vi "NMEA serial.vi"() -> ()   [LabVIEW 2016, in "AIRMAR WeatherCaster.lvlib"]
uses:
  AIRMAR WeatherCaster.lvlib
  NMEA_WIMDA-data.ctl
  NMEA_GPRMC-data.ctl
  NMEA_LatitudeDirection.ctl
  NMEA_LongitudeDirection.ctl
  <vilib>/Utility/miscctls.llb/LVPointTypeDef.ctl
  <vilib>/Instr/_visa.llb/VISA Configure Serial Port (Instr).vi
  <vilib>/ptbypt/NI_PtbyPt.lvlib
panel:
  in  "重新定标":bool
  out "定标位置":cluster{"Latitude":dbl, "Longitude":dbl} {"Longitude" format="%0.4f [long]"; "Latitude" format="%.04f [lat]"}
  out "移位距离":dbl
  in  "移位报警设定值":u32=1000
  out "$GPRMC-message_OUT":T1={"TimeStamp"=timestamp(0 s since 1904-01-01), "Validity"=FALSE, "Latitude"=0.0, "Latitude-Direction"=enum."North", "Longitude"=0.0, "Longitude-Direction"=enum."East", "Speed in knots"=0.0, "True course"=0.0, "Date Stamp"=timestamp(0 s since 1904-01-01), "Magnetic Variation (East/West)"=0.0} {"Magnetic Variation (East/West)" format="%.02f [deg]"; "Date Stamp" format="%<%x>T"; "True course" format="%.02f [deg]"; "Speed in knots" format="%.02f [kts]"; "Longitude" format="%0.4f [long]"; "Latitude" format="%.04f [lat]"; "TimeStamp" format="%<%.2X>T"}
  out "风向_真角":dbl caption="风向"
  out "风速_m/s":dbl caption="风速"
  out "风速_节":dbl caption="风速"
  out "气温_摄氏度":dbl caption="气温"
  out "气压_mbars":dbl caption="气压"
  out "气压_英寸汞柱":dbl caption="气压"
  out "匹配语句":string
  out "$WIMDA-message_OUT":T4
  in  "串口打开":bool
  out "RAW DATA":string
  in  "baud rate (9600)":u32(ring)=4800 caption="波特率" items=["1200"=1200, "2400"=2400, "4800"=4800, "9600"=9600, "38400"=38400, "115200"=115200]
  in  "VISA resource name":refnum<visa-resource-name> caption="串口"
  # "米"
  # "米"
  # "°"
  # "m/s"
  # "节"
  # "℃"
  # "mbars"
  # "英寸汞柱"
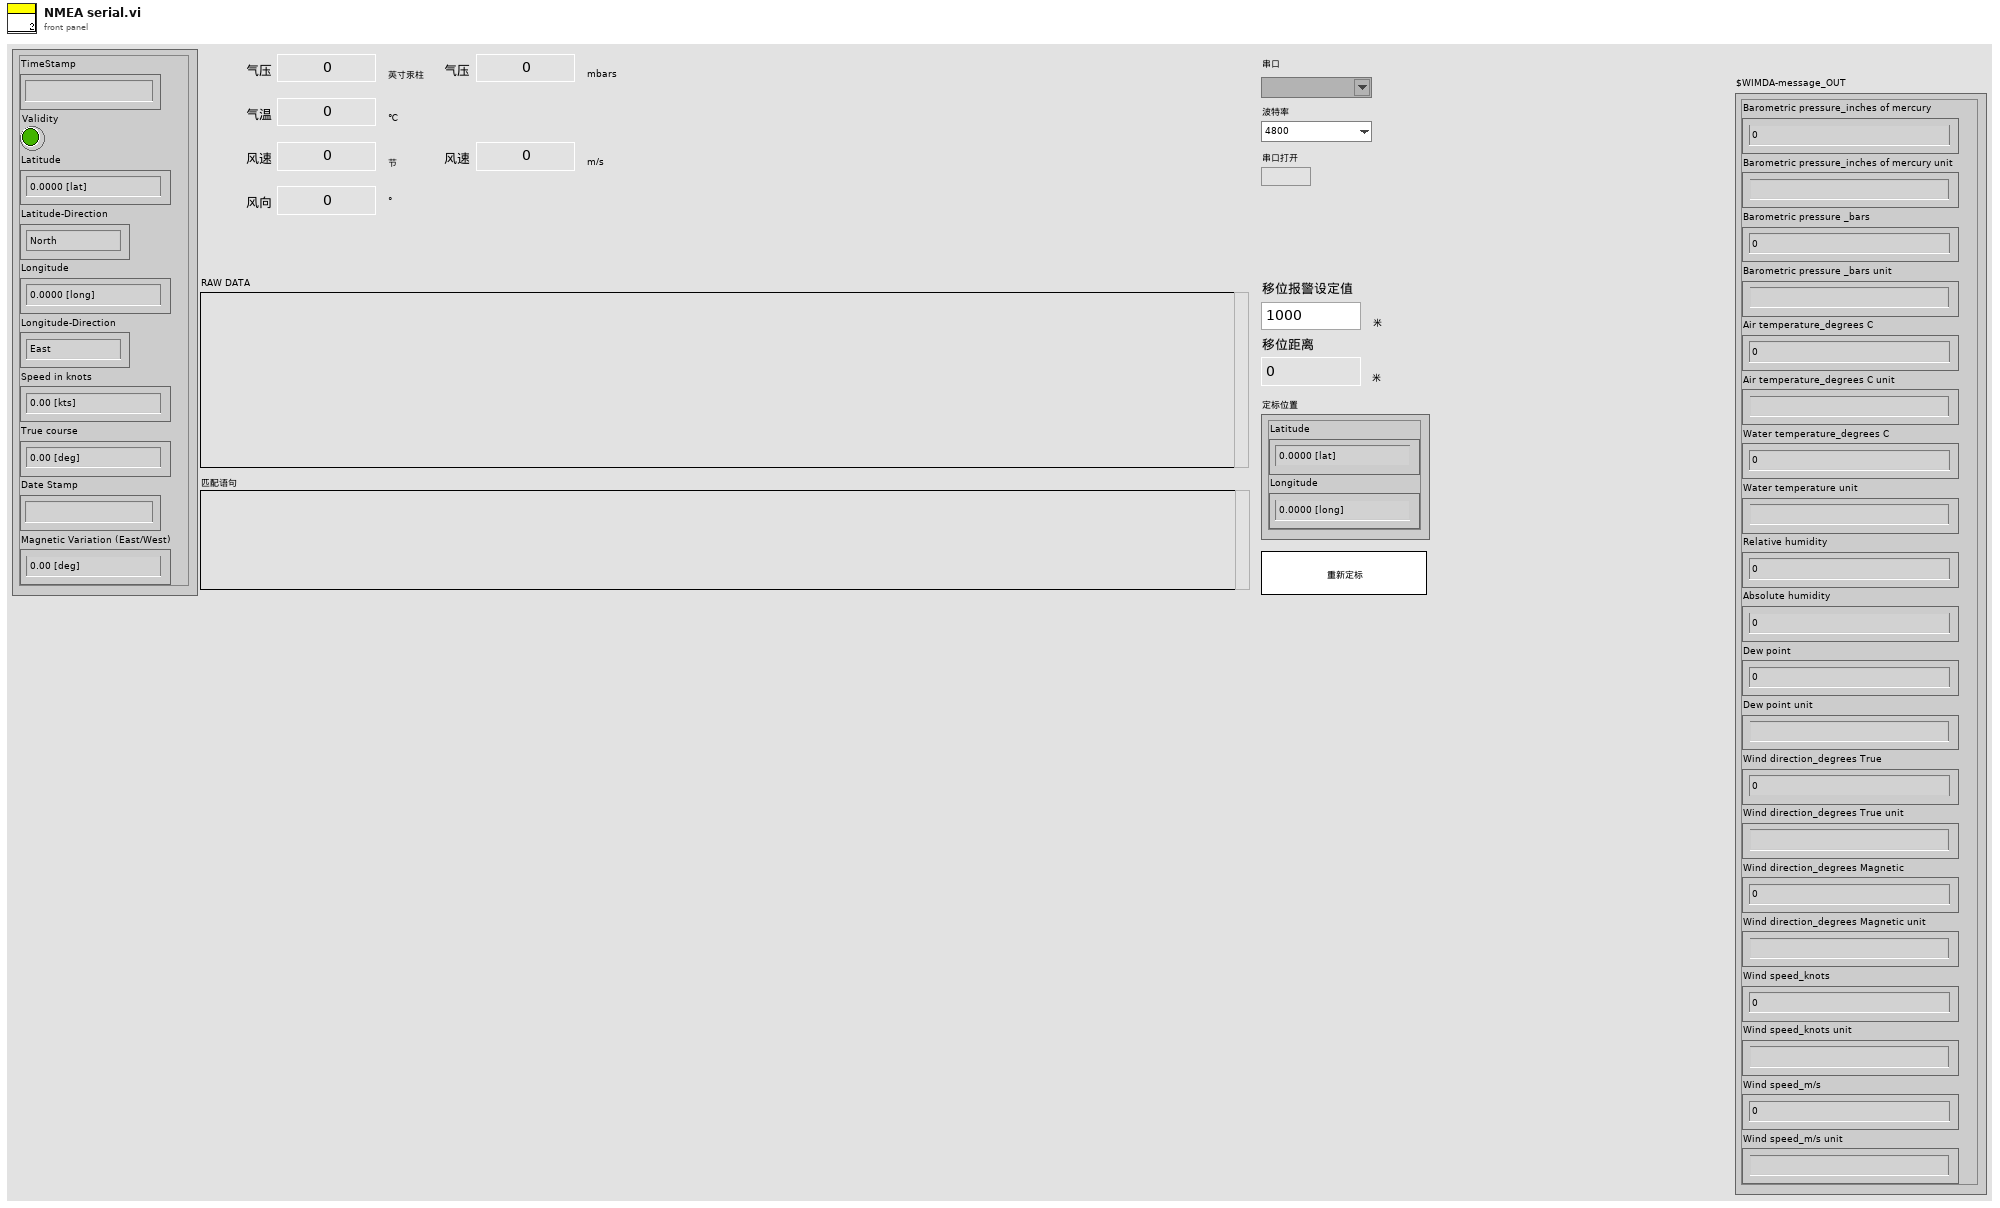
[diagram p1: front panel]
types:
  T1 = typedef "AIRMAR WeatherCaster.lvlib/NMEA_GPRMC-data.ctl" = cluster{"TimeStamp":timestamp, "Validity":bool, "Latitude":dbl, "Latitude-Direction":T2, "Longitude":dbl, "Longitude-Direction":T3, "Speed in knots":dbl, "True course":dbl, "Date Stamp":timestamp, "Magnetic Variation (East/West)":dbl}
  T2 = typedef "AIRMAR WeatherCaster.lvlib/NMEA_LatitudeDirection.ctl" = enum16{"", "North", "South"}
  T3 = typedef "AIRMAR WeatherCaster.lvlib/NMEA_LongitudeDirection.ctl" = enum16{"", "East", "West"}
  T4 = typedef "AIRMAR WeatherCaster.lvlib/NMEA_WIMDA-data.ctl" = cluster{"Barometric pressure_inches of mercury":dbl, "Barometric pressure_inches of mercury unit":string, "Barometric pressure _bars":dbl, "Barometric pressure _bars unit":string, "Air temperature_degrees C":dbl, "Air temperature_degrees C unit":string, "Water temperature_degrees C":dbl, "Water temperature unit":string, "Relative humidity":dbl, "Absolute humidity":dbl, "Dew point":dbl, "Dew point unit":string, "Wind direction_degrees True":dbl, "Wind direction_degrees True unit":string, "Wind direction_degrees Magnetic":dbl, "Wind direction_degrees Magnetic unit":string, "Wind speed_knots":dbl, "Wind speed_knots unit":string, "Wind speed_m/s":dbl, "Wind speed_m/s unit":string}
  T5 = typedef "LVPointTypeDef.ctl" = cluster{"Horizontal":i16, "Vertical":i16}
  T6 = typedef "LVDateTimeRec.ctl" = cluster{"秒数的小数部分":dbl, "秒":i32, "分":i32, "时":i32, "日":i32, "月":i32, "年":i32, "天数（周）":i32, "天数（年）":i32, "DST":i32}
  T7 = cluster{"VISA resource name":refnum<visa-resource-name>, "baud rate (9600)":u32, "串口打开":bool}
  T8 = enum8{"Enabled", "Disabled", "Disabled and Grayed Out"}
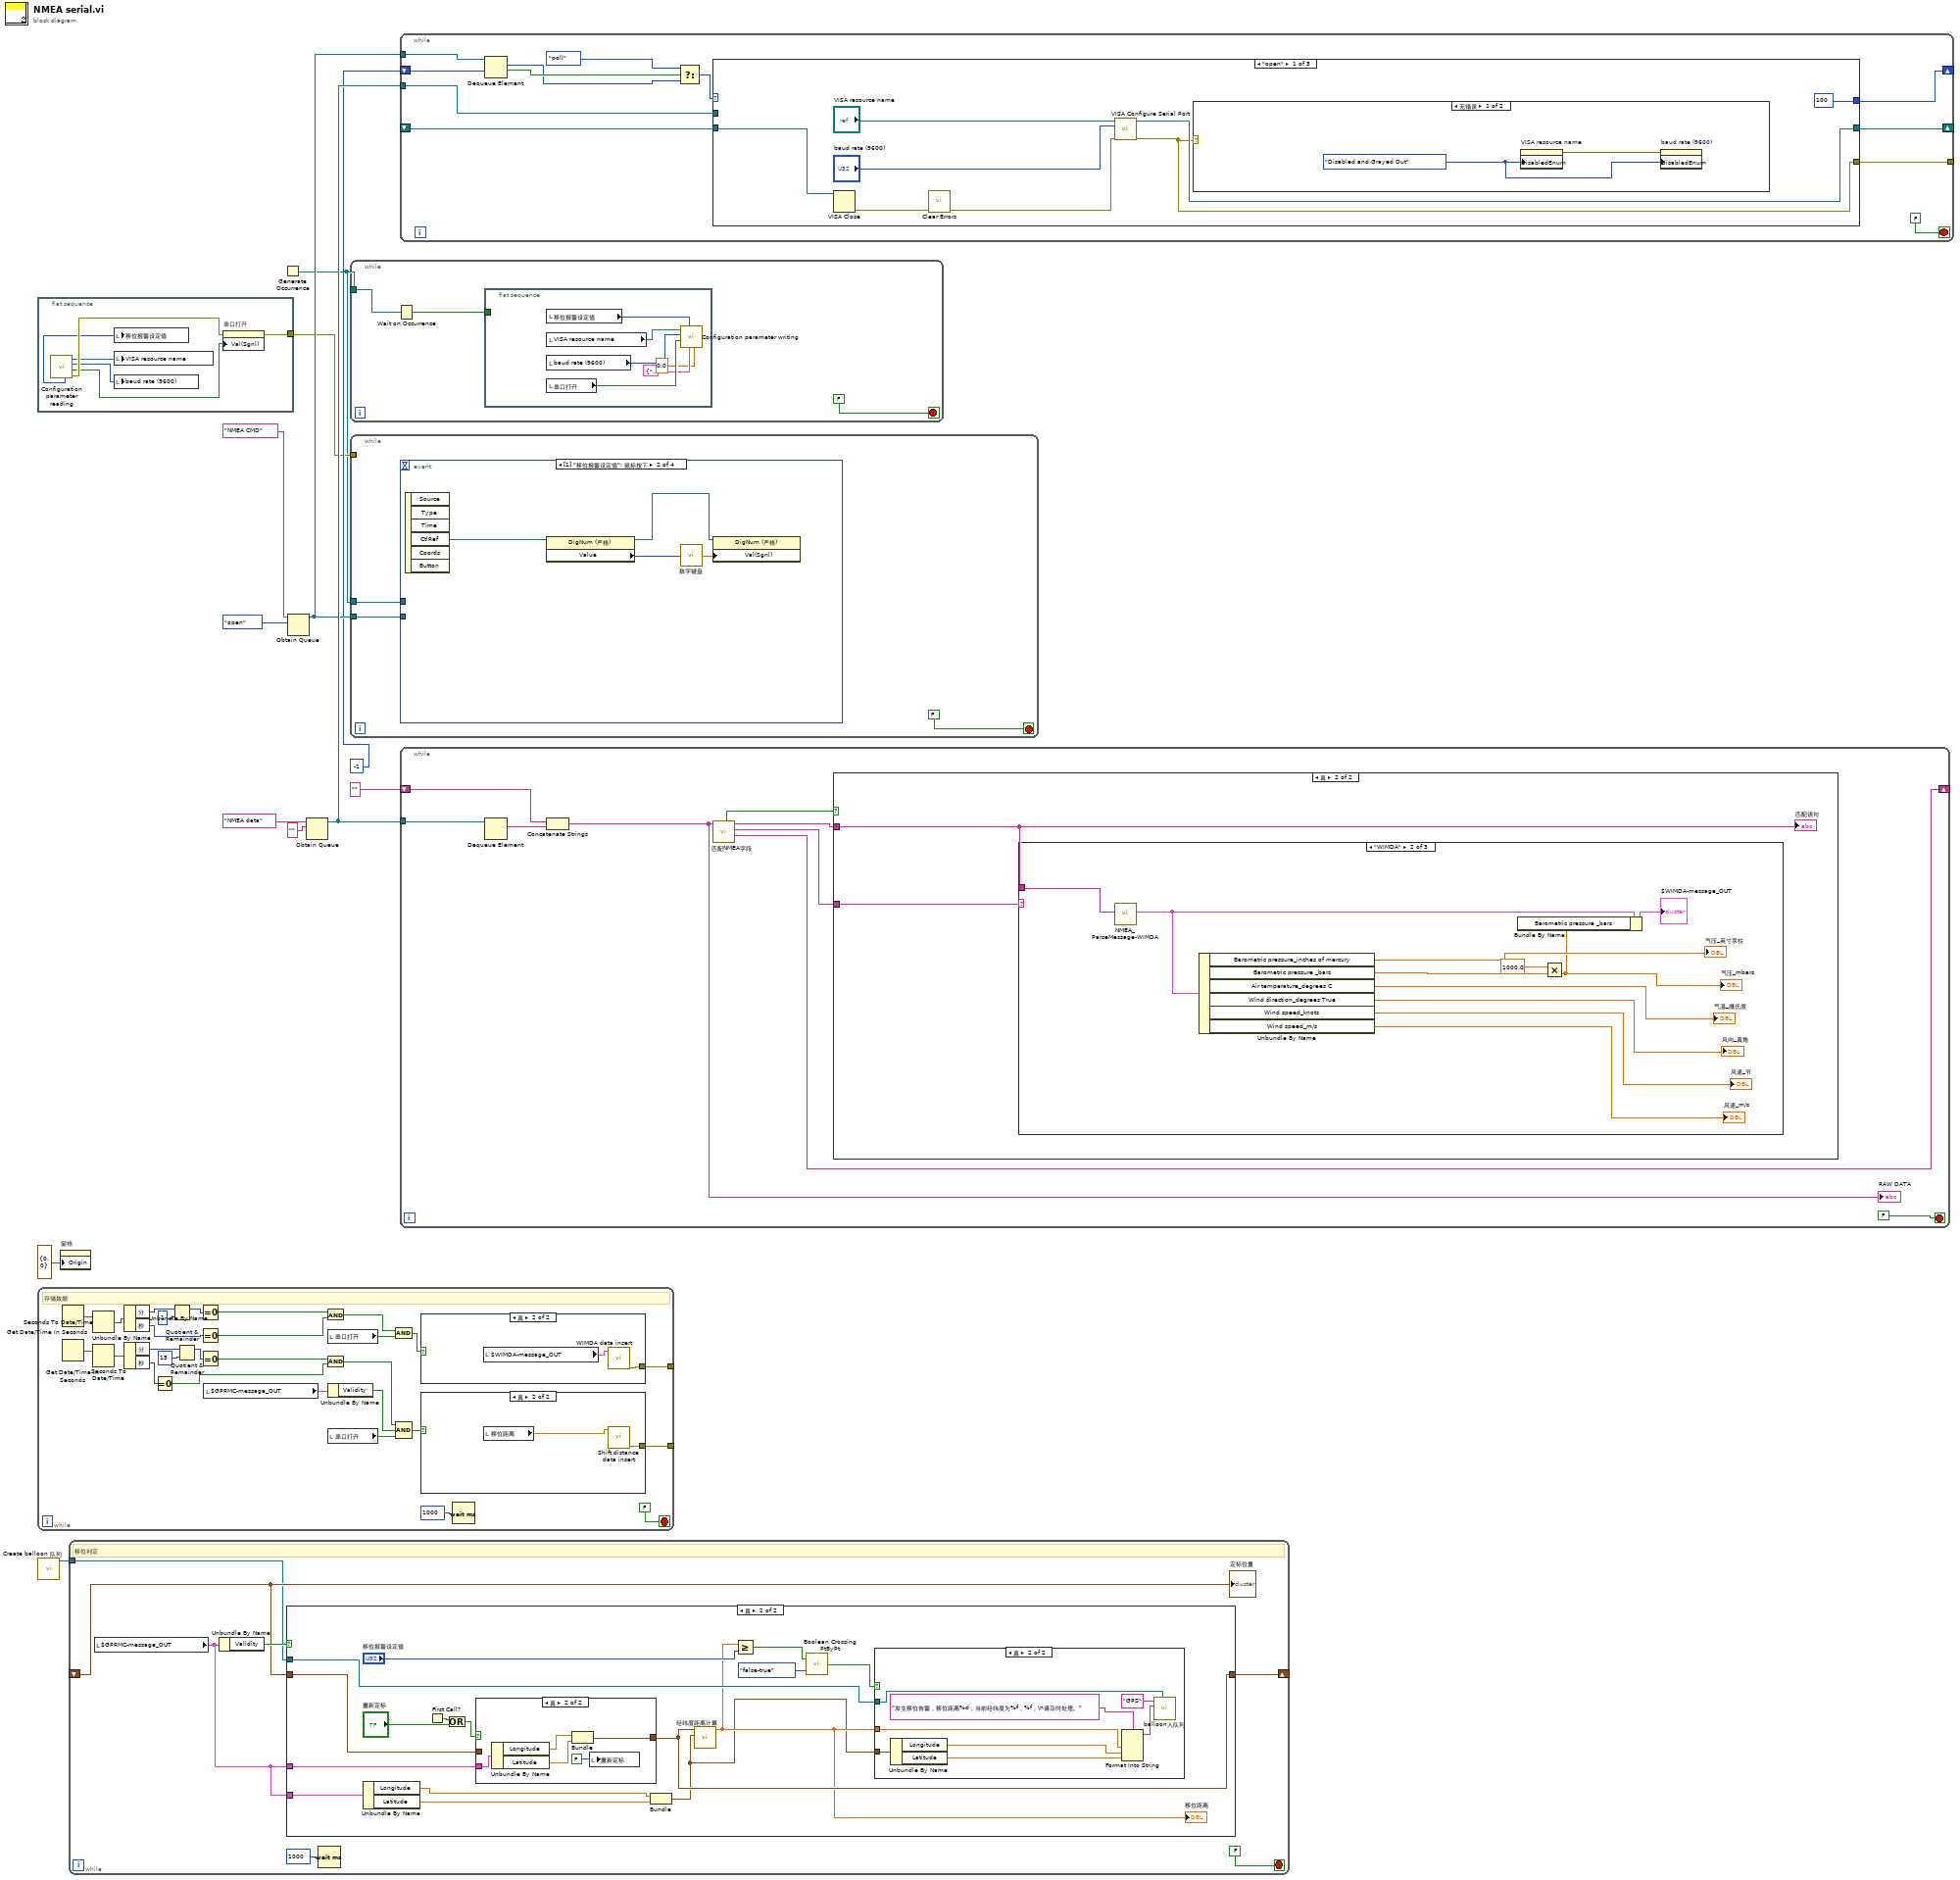
[diagram p0: block diagram]
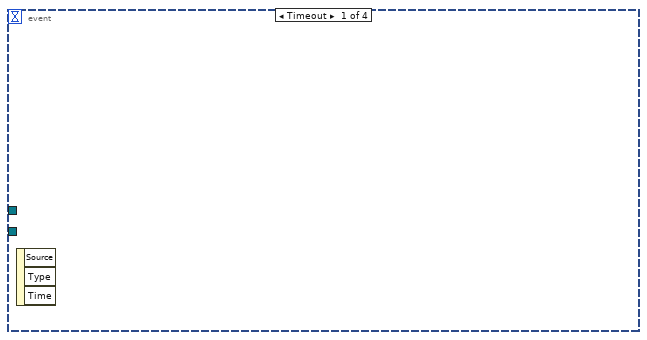
[diagram p7: hidden frame]
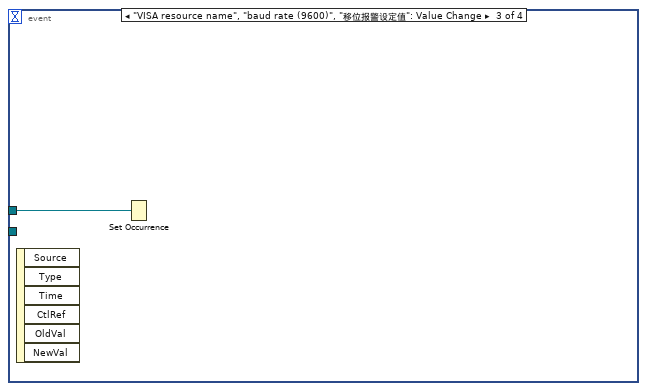
[diagram p8: hidden frame]
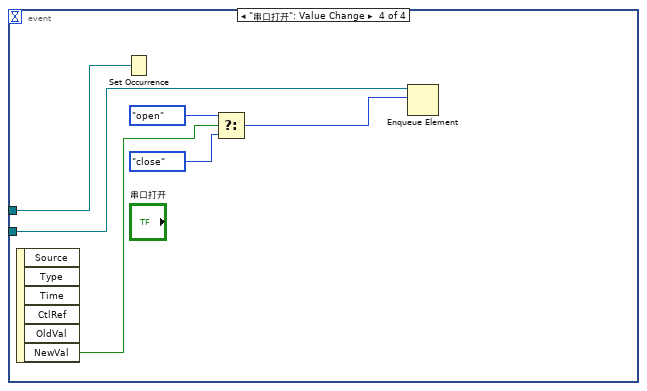
[diagram p9: hidden frame]
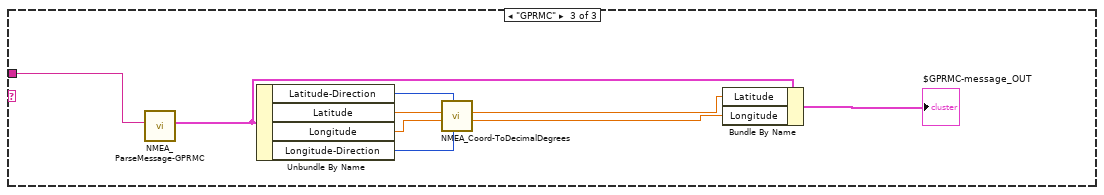
[diagram p12: hidden frame]
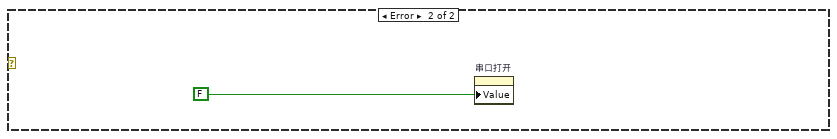
[diagram p13: hidden frame]
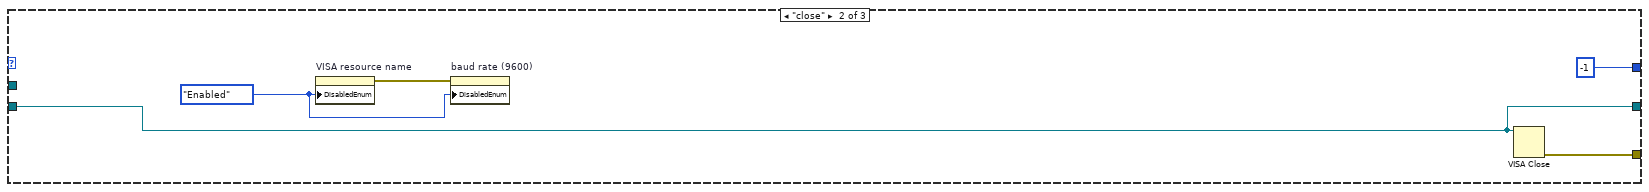
[diagram p14: hidden frame]
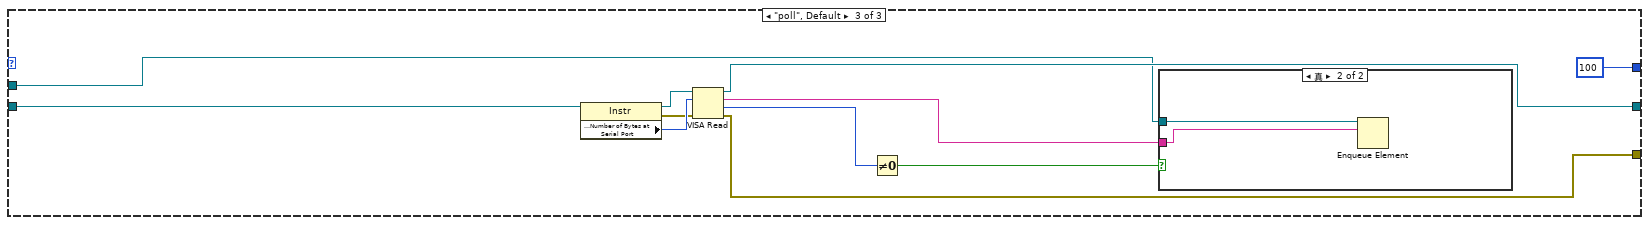
[diagram p15: hidden frame]
diagram:
  n1 = flat-sequence {
    tunnel: [w18] -> w3
    frame #0 {
      n2 = call "Configuration parameter reading.vi"() -> ("error out"=w17:errorcluster, "enable"=w14:bool, "baud rate (9600)"=w16:u32, "VISA resource name"=w15:refnum<visa-resource-name>, "Shift distance"=w13:u32)  [unwired: 5 in, 2 out]
      n3 = local write "移位报警设定值"(w13) -> ()
      n4 = local write "VISA resource name"(w15) -> ()
      n5 = local write "baud rate (9600)"(w16) -> ()
      n6 = property on="串口打开" class="Bool (严格)"(error in=w17, "Val(Sgnl)"=w14) -> (error out=w18:errorcluster)  [unwired: 1 in, 1 out]
    }
  }
  n7 = while {
    tunnel: [w21] -> _
    tunnel: [w20] -> _
    stop <- FALSE stop-if-true
    # "存储数据"
    n8 = Get Date/Time In Seconds() -> (seconds since 1Jan1904=w37:timestamp)
    n9 = Get Date/Time In Seconds() -> (seconds since 1Jan1904=w33:timestamp)
    n10 = Seconds To Date/Time(time stamp (now)=w37) -> (date time rec=w45:T6)  [unwired: 1 in]
    n11 = Seconds To Date/Time(time stamp (now)=w33) -> (date time rec=w25:T6)  [unwired: 1 in]
    n12 = Unbundle By Name(w45) -> ("分"=w44:i32, "秒"=w41:i32)
    n13 = Unbundle By Name(w25) -> ("分"=w26:i32, "秒"=w29:i32)
    n14 = Equal To 0?(x=w29) -> (x = 0?=w31:bool)
    n15 = Quotient & Remainder(x=w44, y=1) -> (x-y*floor(x/y)=w42:i32)  [unwired: 1 out]
    n16 = Quotient & Remainder(x=w26, y=15) -> (x-y*floor(x/y)=w28:i32)  [unwired: 1 out]
    n17 = Equal To 0?(x=w42) -> (x = 0?=w40:bool)
    n18 = Equal To 0?(x=w41) -> (x = 0?=w39:bool)
    n19 = Equal To 0?(x=w28) -> (x = 0?=w30:bool)
    n20 = local read "$GPRMC-message_OUT"() -> (w23:T1)
    n21 = And(x=w40, y=w39) -> (x .and. y?=w38:bool)
    n22 = And(x=w30, y=w31) -> (x .and. y?=w32:bool)
    n23 = local read "串口打开"() -> (w34:bool)
    n24 = Unbundle By Name(w23) -> ("Validity"=w22:bool)
    n25 = local read "串口打开"() -> (w19:bool)
    n26 = And(x=w38, y=w34) -> (x .and. y?=w35:bool)
    n27 = Compound Arithmetic op=AND ("复合运算")(w32, w22, w19) -> (w24:bool)
    n28 = case shown="真" w35 {
      tunnel: [_ w49] -> w21
      frame False {
      }
      frame True {
        n29 = local read "$WIMDA-message_OUT"() -> (w50:T4)
        n30 = call "WIMDA data insert.vi"("WIMDA-data"=w50) -> ("error out"=w49:errorcluster)  [unwired: 10 in]
      }
    }
    n31 = case shown="真" w24 {
      tunnel: [_ w48] -> w20
      frame False {
      }
      frame True {
        n32 = local read "移位距离"() -> (w47:dbl)
        n33 = call "Shift distance data insert.vi"("移位距离"=w47) -> ("error out"=w48:errorcluster)  [unwired: 10 in]
      }
    }
    n34 = Wait (ms)(milliseconds to wait=u32 1000 ("等待时间（毫秒）")) -> ()  [unwired: 1 out]
  }
  n35 = call "Create balloon 队列.vi"() -> ("队列输出"=w1:refnum<queue>)  [unwired: 11 in]
  n36 = property on="窗格" class="Pane"("Origin"=T5 {"Horizontal"=0, "Vertical"=0} ("原点")) -> ()  [unwired: 2 in, 2 out]
  n37 = while {
    shift-right: [w57] -> _
    shift-left: _ -> [w53]
    tunnel: w1 -> [w51]
    stop <- FALSE stop-if-true
    # "移位判定"
    n38 = local read "$GPRMC-message_OUT"() -> (w54:T1)
    n39 = Unbundle By Name(w54) -> ("Validity"=w55:bool)
    n40 = case shown="真" w55 {
      tunnel: [w58 w72] -> w57
      tunnel: w53 -> [w58 w71]
      tunnel: w54 -> [_ w70]
      tunnel: w54 -> [_ w69]
      tunnel: w51 -> [_ w65]
      frame False {
      }
      frame True {
        n41 = Unbundle By Name(w69) -> ("Longitude"=w74:dbl, "Latitude"=w73:dbl)
        n42 = First Call?() -> (First Call?: T/F=w68:bool)
        n43 = Or(x=w68, y="重新定标") -> (x .or. y?=w67:bool)
        n44 = case shown="真" w67 {
          tunnel: [w83 w86] -> w72
          tunnel: w71 -> [w83 _]
          tunnel: w70 -> [_ w85]
          frame False {
          }
          frame True {
            n45 = Unbundle By Name(w85) -> ("Longitude"=w87:dbl, "Latitude"=w88:dbl)
            n46 = Bundle("Longitude"=w87, "Latitude"=w88) -> (w86:cluster{"Longitude":dbl, "Latitude":dbl})  [unwired: 1 in]
            n47 = local write "重新定标"(FALSE ("重新定标")) -> ()
          }
        }
        n48 = Bundle("Longitude"=w74, "Latitude"=w73) -> (w59:cluster{"Longitude":dbl, "Latitude":dbl})  [unwired: 1 in]
        n49 = call "经纬度距离计算.vi"("结束位置"=w59, "起始位置"=w72) -> ("距离"=w60:dbl)  [unwired: 9 in]
        "移位距离" <- w60
        n50 = Greater Or Equal?(x=w60, y="移位报警设定值") -> (x >= y?=w63:bool)
        n51 = call <vilib>:"Boolean Crossing PtByPt.vi"("direction"=enum16{"either", "false-true", "true-false"}."false-true", "input"=w63) -> ("crossing"=w61:bool)  [unwired: 1 in]
        n52 = case shown="真" w61 {
          tunnel: w65 -> [_ w82]
          tunnel: w60 -> [_ w78]
          tunnel: w59 -> [_ w77]
          frame False {
          }
          frame True {
            n53 = Unbundle By Name(w77) -> ("Longitude"=w76:dbl, "Latitude"=w75:dbl)
            n54 = Format Into String(format string="发生移位告警，移位距离%d，当前经纬度为%f，%f；\n请及时处理。" ("格式字符串"), w78, w76, w75) -> (resulting string=w79:string)  [unwired: 2 in, 1 out]
            n55 = call "balloon入队列.vi"("队列"=w82, "故障信息"=w79, "参数名称"="GPS") -> ()  [unwired: 8 in, 1 out]
          }
        }
      }
    }
    n56 = Wait (ms)(milliseconds to wait=u32 1000 ("等待时间（毫秒）")) -> ()  [unwired: 1 out]
    "定标位置" <- w53
  }
  n57 = Generate Occurrence() -> (w2:refnum<k4>)
  n58 = Obtain Queue(name (unnamed)="NMEA CMD" ("名称（未命名）"), element data type=enum16{"open", "close", "poll"}."open" ("枚举")) -> (queue out=w6:refnum<queue>)  [unwired: 3 in, 2 out]
  n59 = Obtain Queue(name (unnamed)="NMEA data" ("名称（未命名）"), element data type="") -> (queue out=w8:refnum<queue>)  [unwired: 3 in, 2 out]
  n60 = while {
    tunnel: w2 -> [w90]
    stop <- FALSE stop-if-true
    n61 = Wait on Occurrence(2:w90) -> (0:w89:bool)  [unwired: 2 in]
    n62 = flat-sequence {
      tunnel: w89 -> [_]
      frame #0 {
        n63 = local read "移位报警设定值"() -> (w94:u32)
        n64 = local read "VISA resource name"() -> (w97:refnum<visa-resource-name>)
        n65 = local read "baud rate (9600)"() -> (w96:u32)
        n66 = local read "串口打开"() -> (w95:bool)
        n67 = call "Configuration parameter writing.vi"("Calibration angle"=sgl 0.0, "电子罗盘"=T7 {"VISA resource name"="", "baud rate (9600)"=9600, "串口打开"=FALSE}, "Shift distance"=w94, "enable"=w95, "baud rate (9600)"=w96, "VISA resource name"=w97) -> ()  [unwired: 5 in, 1 out]
      }
    }
  }
  n68 = while {
    tunnel: w6 -> [w99]
    tunnel: w3 -> [_]
    tunnel: w2 -> [w98]
    stop <- FALSE stop-if-true
    n69 = event shown="[1] \"移位报警设定值\": 鼠标按下" {
      selector: _ -> [_ _ _ _]
      dyn-events: _ -> [_ _ _ _]
      timeout: _ -> [_ _ _ _]
      tunnel: w99 -> [_ _ _ w111]
      tunnel: w98 -> [_ _ w105 w106]
      event Timeout {
        n70 = event-data() -> ()  [unwired: 1 in, 3 out]
      }
      event "移位报警设定值": Mouse Down {
        n71 = event-data() -> ("CtlRef"=w104:refnum<vi>)  [unwired: 1 in, 5 out]
        n72 = property class="DigNum (严格)"(reference=w104) -> (reference out=w103:refnum<vi>, "Value"=w102:u32)  [unwired: 1 in, 1 out]
        n73 = call "数字键盘.vi"("OldNumber"=w102) -> ("NewNumber"=w101:sgl)
        n74 = property class="DigNum (严格)"(reference=w103, "Val(Sgnl)"=w101) -> ()  [unwired: 1 in, 2 out]
      }
      event "VISA resource name", "baud rate (9600)", "移位报警设定值": Value Change {
        n75 = event-data() -> ()  [unwired: 1 in, 6 out]
        n76 = Set Occurrence(w105) -> ()
      }
      event "串口打开": Value Change {
        n77 = event-data() -> ("NewVal"=w110:bool)  [unwired: 1 in, 5 out]
        n78 = Set Occurrence(w106) -> ()
        n79 = Select(t=enum16{"open", "close", "poll"}."open" ("元素"), s=w110, f=enum16{"open", "close", "poll"}."close") -> (s? t:f=w108:enum16{"open", "close", "poll"})
        n80 = Enqueue Element(queue=w111, element=w108) -> ()  [unwired: 2 in, 3 out]
      }
    }
  }
  n81 = while {
    shift-right: [w123] -> _
    shift-left: _ -> [w122]
    tunnel: w6 -> [w121]
    tunnel: [w120] -> _
    tunnel: w8 -> [w119]
    shift-right: [w112] -> _
    shift-left: -1 ("超时毫秒(-1)") -> [w113]
    stop <- FALSE stop-if-true
    n82 = Dequeue Element(queue=w121, timeout in ms (-1)=w113) -> (element=w115:enum16{"open", "close", "poll"}, timed out?=w117:bool)  [unwired: 1 in, 2 out]
    n83 = Select(t=enum16{"open", "close", "poll"}."poll" ("枚举"), s=w117, f=w115) -> (s? t:f=w114:enum16{"open", "close", "poll"})
    n84 = case shown="\"open\"" w114 {
      tunnel: [w129 w139 w150] -> w123
      tunnel: w122 -> [w128 w139 w148]
      tunnel: [w124 w138 w149] -> w120
      tunnel: w119 -> [_ _ w145]
      tunnel: [100 ("超时毫秒(-1)") -1 ("超时毫秒(-1)") 100 ("超时毫秒(-1)")] -> w112
      frame "open" {
        n85 = VISA Close(VISA resource name=w128) -> (error out=w127:errorcluster)  [unwired: 1 in]
        n86 = call <vilib>:"Clear Errors.vi"("error in (no error)"=w127) -> ("error out"=w126:errorcluster)  [unwired: 5 in, 1 out]
        n87 = call-poly "VISA Configure Serial Port"("VISA resource name"="VISA resource name", "baud rate (9600)"="baud rate (9600)", "error in (no error)"=w126) -> ("VISA resource name out"=w129:refnum<visa-resource-name>, "error out"=w124:errorcluster)  [unwired: 11 in]
        n88 = case shown="无错误" w124 {
          frame No Error {
            w133 = T8."Disabled and Grayed Out" ("禁用")
            n89 = property on="VISA resource name" class="VISAName"("DisabledEnum"=w133) -> (error out=w132:errorcluster)  [unwired: 2 in, 1 out]
            n90 = property on="baud rate (9600)" class="Ring (严格)"(error in=w132, "DisabledEnum"=w133) -> ()  [unwired: 1 in, 2 out]
          }
          frame Error {
            n91 = property on="串口打开" class="Bool (严格)"("Value"=FALSE ("串口打开")) -> ()  [unwired: 2 in, 2 out]
          }
        }
      }
      frame "close" {
        w135 = T8."Enabled" ("禁用")
        n92 = property on="VISA resource name" class="VISAName"("DisabledEnum"=w135) -> (error out=w136:errorcluster)  [unwired: 2 in, 1 out]
        n93 = property on="baud rate (9600)" class="Ring (严格)"(error in=w136, "DisabledEnum"=w135) -> ()  [unwired: 1 in, 2 out]
        n94 = VISA Close(VISA resource name=w139) -> (error out=w138:errorcluster)  [unwired: 1 in]
      }
      frame "poll", Default {
        n95 = property class="Instr"(reference=w148) -> (reference out=w147:refnum<visa-resource-name>, error out=w141:errorcluster, "Serial Settings:Number of Bytes at Serial Port"=w146:u32)  [unwired: 1 in]
        n96 = VISA Read(VISA resource name=w147, byte count=w146, error in (no error)=w141) -> (VISA resource name out=w150:refnum<visa-resource-name>, read buffer=w144:string, return count=w143:u32, error out=w149:errorcluster)
        n97 = Not Equal To 0?(x=w143) -> (x != 0?=w142:bool)
        n98 = case shown="真" w142 {
          tunnel: w145 -> [_ w152]
          tunnel: w144 -> [_ w151]
          frame False {
          }
          frame True {
            n99 = Enqueue Element(queue=w152, element=w151) -> ()  [unwired: 2 in, 3 out]
          }
        }
      }
    }
  }
  n100 = while {
    tunnel: w8 -> [w161]
    shift-right: [w154] -> _
    shift-left: "" -> [w159]
    stop <- FALSE stop-if-true
    n101 = Dequeue Element(queue=w161) -> (element=w160:string)  [unwired: 2 in, 3 out]
    n102 = Concatenate Strings(w159, w160) -> (w157:string)
    "RAW DATA" <- w157
    n103 = call "匹配NMEA字段.vi"("输入字符串"=w157) -> ("未匹配语句"=w154:string, "NMEA语句"=w153:string, "匹配语句"=w156:string, "匹配"=w155:bool)  [unwired: 7 in]
    n104 = case shown="真" w155 {
      tunnel: w156 -> [_ w163]
      tunnel: w153 -> [_ w162]
      frame False {
      }
      frame True {
        n105 = case shown="\"WIMDA\"" w162 {
          tunnel: w163 -> [_ w174 w183]
          frame "假", Default {
          }
          frame "WIMDA" {
            n106 = call "NMEA_ParseMessage-WIMDA.vi"("$WIMDA-message_IN"=w174) -> ("$WIMDA-message_OUT"=w173:T4)  [unwired: 9 in, 1 out]
            n107 = Unbundle By Name(w173) -> ("Barometric pressure_inches of mercury"=→"气压_英寸汞柱":dbl, "Barometric pressure _bars"=w171:dbl, "Air temperature_degrees C"=→"气温_摄氏度":dbl, "Wind direction_degrees True"=→"风向_真角":dbl, "Wind speed_knots"=→"风速_节":dbl, "Wind speed_m/s"=→"风速_m/s":dbl)
            n108 = Multiply(x=1000.0, y=w171) -> (x*y=w164:dbl)
            "气压_mbars" <- w164
            n109 = Bundle By Name(cluster=w173, "Barometric pressure _bars"=w164) -> (→"$WIMDA-message_OUT":T4)
          }
          frame "GPRMC" {
            n110 = call "NMEA_ParseMessage-GPRMC.vi"("$GPRMC-message_IN"=w183) -> ("$GPRMC-message_OUT"=w182:T1)  [unwired: 9 in, 1 out]
            n111 = Unbundle By Name(w182) -> ("Latitude-Direction"=w178:T2, "Latitude"=w181:dbl, "Longitude"=w180:dbl, "Longitude-Direction"=w179:T3)
            n112 = call "NMEA_Coord-ToDecimalDegrees.vi"("Longitude-Direction"=w179, "Latitude-Direction"=w178, "Longitude"=w180, "Latitude"=w181) -> ("Longitude"=w175:dbl, "Latitude"=w176:dbl)  [unwired: 6 in]
            n113 = Bundle By Name(cluster=w182, "Latitude"=w176, "Longitude"=w175) -> (→"$GPRMC-message_OUT":T1)
          }
        }
        "匹配语句" <- w163
      }
    }
  }
